vi "Sweep Dictionary.vi"(0 "Sweep name":string, 5 "Action":T1, 9 "Sweep in":variant) -> (4 "Sweep out":variant, 6 "Sweep not found / already included":bool, 10 "All sweeps out":variant[](array[variant]))   [LabVIEW 2023, in "RFCalAndFixtureCharact.Common.lvlib"]
uses:
  RFCalAndFixtureCharact.Common.lvlib
  Type Definitions/Dictionary Operation.ctl
  <vilib>/Utility/miscctls.llb/LVMapReplaceAction.ctl
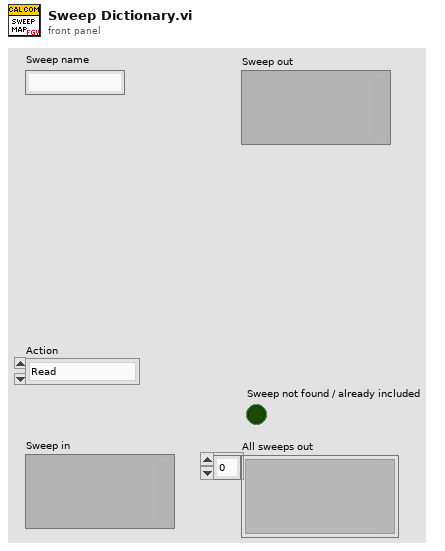
[diagram p1: front panel]
types:
  T1 = typedef "RFCalAndFixtureCharact.Common.lvlib/Dictionary Operation.ctl" = enum16{"Read", "Insert", "Remove", "Clear", "Get All", "Update"}
  T2 = typedef "LVMapReplaceAction.ctl" = enum32{"Modify Entry only if found", "Add or Modify Entry", "Delete Entry"}
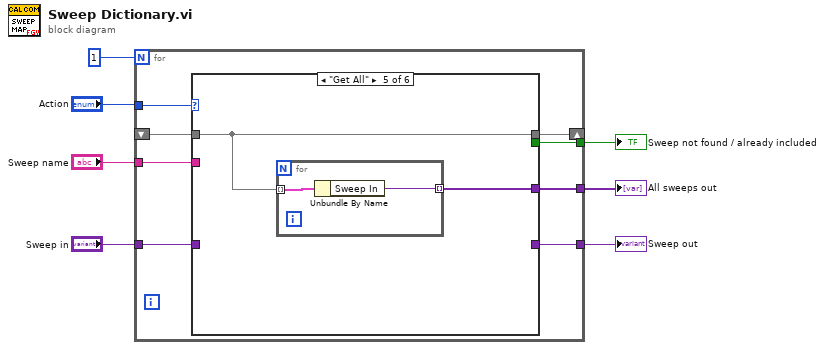
[diagram p0: block diagram]
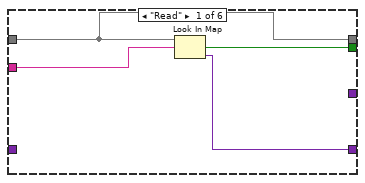
[diagram p2: hidden frame]
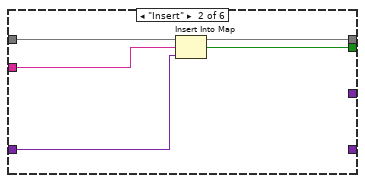
[diagram p3: hidden frame]
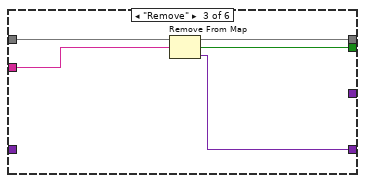
[diagram p4: hidden frame]
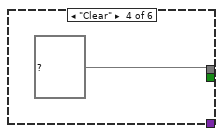
[diagram p5: hidden frame]
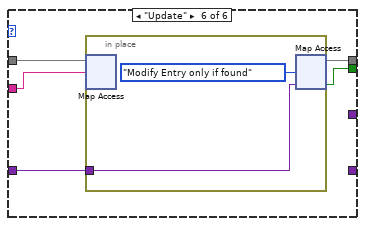
[diagram p6: hidden frame]
diagram:
  n1 = for {
    N: 1 -> [_]
    tunnel: "Action" -> [w15]
    tunnel: "Sweep name" -> [w14]
    tunnel: [w13] -> w5
    tunnel: [w12] -> w1
    shift-right: [w10] -> _
    shift-left: _ -> [w11]
    tunnel: "Sweep in" -> [w9]
    tunnel: [w8] -> w2
    n2 = case shown="\"Get All\"" w15 {
      tunnel: w14 -> [w19 w24 w27 _ _ w39]
      tunnel: w11 -> [w17 w23 w28 _ w32 w35]
      tunnel: [w18 w22 w29 _ _ w36] -> w13
      tunnel: [w16 _ w25 _ _ _] -> w12
      tunnel: [w17 w21 w26 map{string, variant} {} ("Map") w32 w37] -> w10
      tunnel: w9 -> [_ w20 _ _ _ w38]
      tunnel: [_ _ _ _ w31 _] -> w8
      frame "Read" {
        n3 = Look In Map(map=w17, key=w19) -> (key not found?=w18:bool, value=w16:variant)  [unwired: 1 in]
      }
      frame "Insert" {
        n4 = Insert Into Map(map in=w23, key=w24, value=w20) -> (map out=w21:map{string, variant}, key already included?=w22:bool)  [unwired: 1 out]
      }
      frame "Remove" {
        n5 = Remove From Map(10:w27, 11:w28) -> (1:w25:variant, 2:w29:bool, 3:w26:map{string, variant})
      }
      frame "Clear" {
      }
      frame "Get All" {
        n6 = for {
          tunnel: w32 -> [w34] mode=indexing
          tunnel: [w33] -> w31 mode=indexing
          n7 = Unbundle By Name(w34) -> ("Sweep In"=w33:variant)
        }
      }
      frame "Update" {
        n8 = in-place {
          in-place-border: w38 -> [w40]
          n9 = in-place-map #1(w35, w39) -> ()  [unwired: 1 in, 2 out]
          n10 = in-place-map #1(w40, LVMapReplaceAction."Modify Entry only if found" ("action")) -> (w37:map{string, variant}, w36:bool)  [unwired: 1 out]
        }
      }
    }
  }
  "Sweep not found / already included" <- w5
  "All sweeps out" <- w2
  "Sweep out" <- w1
